vi "Line Detector Crop Region.vi"(6 "Region width":dbl=500000.0 format="%#_6pHz", 7 "Frequency":dbl[](array[numeric]), 9 "Magnitude":dbl[](array[numeric]), 10 "Signal":cdb[](array[numeric]), 11 "Center frequency":dbl=500000.0 format="%#_6pHz") -> (1 "Magnitude out":dbl[](array[numeric]), 2 "Signal  out":cdb[](array[numeric]), 3 "Start index":i32, 5 "Frequency out":dbl[](array[numeric]))   [LabVIEW 2016]
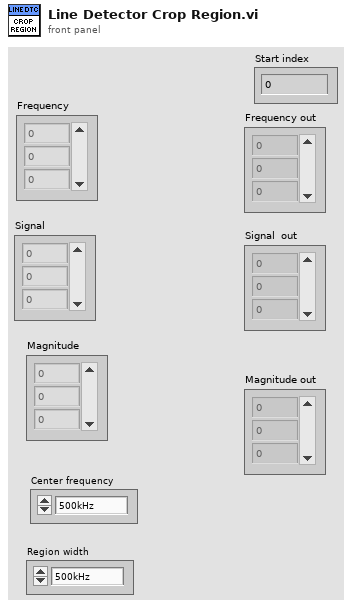
[diagram p1: front panel]
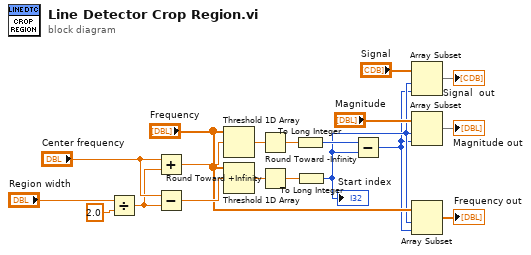
[diagram p0: block diagram]
diagram:
  n1 = Divide(x="Region width", y=2.0) -> (x/y=w14:dbl)
  n2 = Add(x="Center frequency", y=w14) -> (x+y=w7:dbl)
  n3 = Subtract(x="Center frequency", y=w14) -> (x-y=w8:dbl)
  n4 = Threshold 1D Array(2:w7, 3:"Frequency") -> (0:w10:dbl)  [unwired: 1 in]
  n5 = Threshold 1D Array(2:w8, 3:"Frequency") -> (0:w9:dbl)  [unwired: 1 in]
  n6 = Round Toward -Infinity(1:w10) -> (0:w12:dbl)
  n7 = Round Toward +Infinity(x=w9) -> (ceil(x): smallest int >= x=w11:dbl)
  n8 = To Long Integer(number=w12) -> (32bit integer=w13:i32)
  n9 = To Long Integer(number=w11) -> (32bit integer=w3:i32)
  "Start index" <- w3
  n10 = Subtract(x=w13, y=w3) -> (x-y=w2:i32)
  n11 = Array Subset(array="Signal", index=w3, length=w2) -> (→"Signal  out":cdb[])
  n12 = Array Subset(array="Magnitude", index=w3, length=w2) -> (→"Magnitude out":dbl[])
  n13 = Array Subset(array="Frequency", index=w3, length=w2) -> (→"Frequency out":dbl[])
